vi "task5.vi"() -> ()   [LabVIEW 2017]
panel:
  in  "Boolean 7":bool
  in  "Boolean 6":bool
  in  "Boolean 5":bool
  in  "Boolean 4":bool
  in  "Boolean 3":bool
  in  "Boolean 2":bool
  in  "Boolean":bool
  in  "Boolean":bool
  out "Tank":dbl(slide) scale=0.0..255.0
  out "Slide":u8(slide) scale=0.0..255.0
  out "Meter":u32(knob) max=255 scale=0.0..255.0
  in  "stop":bool
  out "Thermometer":dbl(slide) scale=0.0..255.0
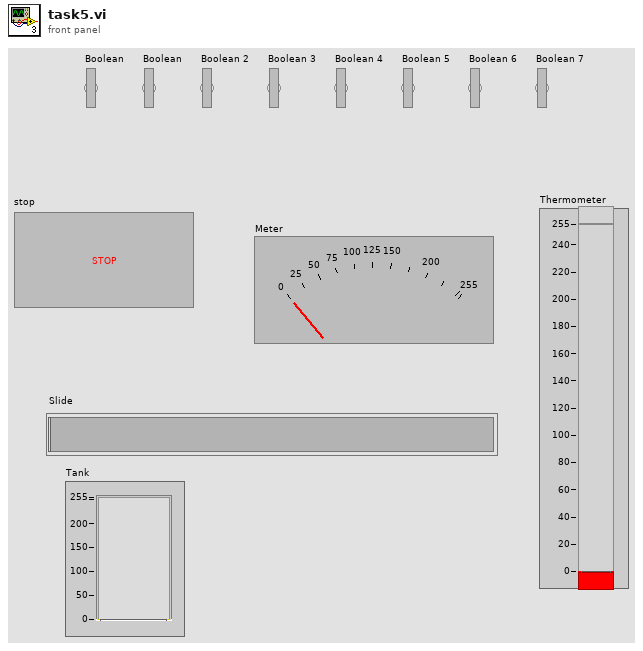
[diagram p1: front panel]
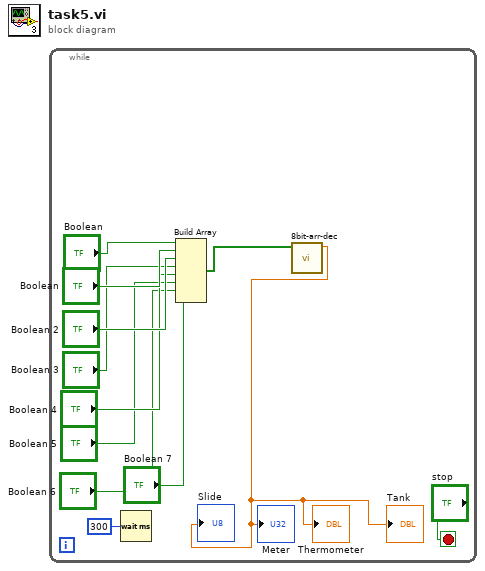
[diagram p0: block diagram]
diagram:
  n1 = while {
    stop <- "stop" stop-if-true
    n2 = Wait (ms)(milliseconds to wait=u32 300) -> ()  [unwired: 1 out]
    n3 = Build Array("Boolean", "Boolean", "Boolean 2", "Boolean 3", "Boolean 4", "Boolean 5", "Boolean 6", "Boolean 7") -> (w2:bool[])
    n4 = call "8bit-arr-dec.vi"("Array"=w2) -> ("f"=→"Thermometer" →"Meter" →"Slide" →"Tank":dbl)  [unwired: 10 in]
  }
